vi "setWavelength.vi"(8 "error in (no error)":errorcluster, 10 "wavelength":T1, 11 "Monochromator in":refnum<class "Monochromator.lvclass">) -> (0 "error out":errorcluster, 2 "IsBusy":bool, 3 "Monochromator out":refnum<class "Monochromator.lvclass">)   [LabVIEW 2016, in "Monochromator.lvclass"]
uses:
  Monochromator.lvclass
  Typedefs/wavelength.ctl
  Monochromator.lvclass/Monochromator.ctl
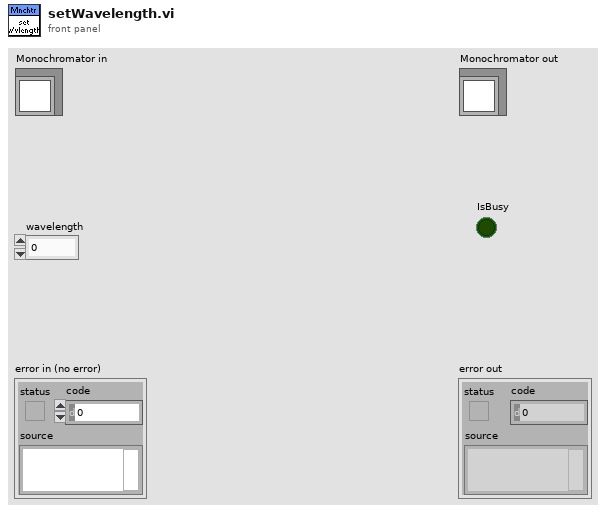
[diagram p1: front panel]
types:
  T1 = typedef "wavelength.ctl" = dbl
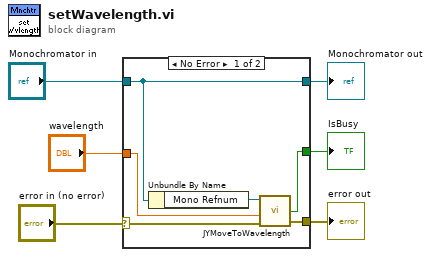
[diagram p0: block diagram]
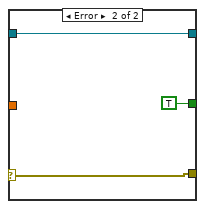
[diagram p2: hidden frame]
diagram:
  n1 = case shown="No Error" "error in (no error)" {
    selector: "error in (no error)" -> [w10 w15]
    tunnel: [w9 w15] -> w5
    tunnel: [w12 w14] -> w3
    tunnel: "Monochromator in" -> [w12 w14]
    tunnel: "wavelength" -> [w7 _]
    tunnel: [w8 TRUE ("IsBusy")] -> w1
    frame No Error {
      n2 = Unbundle By Name(w12) -> ("Mono Refnum"=w11:refnum<k7>)
      n3 = call "JYMoveToWavelength.vi"("error in (no error)"=w10, "Target WL"=w7, "RefNum In"=w11) -> ("error out"=w9:errorcluster, "IsBusy"=w8:bool)  [unwired: 1 in, 1 out]
    }
    frame Error {
    }
  }
  "error out" <- w5
  "Monochromator out" <- w3
  "IsBusy" <- w1
